vi "test13-Broadcast_Event.vi"(8 "error in (no error)":errorcluster, 11 "TestCase in":refnum<class "testcase-CSMGlobalLog.lvclass">) -> (0 "error out":errorcluster, 3 "TestCase out":refnum<class "testcase-CSMGlobalLog.lvclass">)   [LabVIEW 2017, in "testcase-CSMGlobalLog.lvclass"]
uses:
  testcase-CSMGlobalLog.lvclass
  testcase-CSMGlobalLog.lvclass/testcase-CSMGlobalLog.ctl
  src/user.lib/_NEVSTOP/Communicable State Machine(CSM)/_Support/Typedef/_CSM_GlobalLog_MSG.ctl
  src/user.lib/_NEVSTOP/Communicable State Machine(CSM)/_Support/Typedef/_CSM_Response Source Message.ctl
  src/user.lib/_NEVSTOP/Communicable State Machine(CSM)/_Support/Typedef/_CSM_GlobalLog_MSG_TYPE.ctl
  c0dc643a-0362-49fc-99f4-5251266ba5a0.vi
  src/user.lib/_NEVSTOP/Communicable State Machine(CSM)/_Support/GlobalEvent/GEvt-Generate with Rule Check.vi
  src/user.lib/_NEVSTOP/Communicable State Machine(CSM)/AdvanceAPI/CSM - Convert Error to Argument.vi
  src/user.lib/_NEVSTOP/Communicable State Machine(CSM)/AdvanceAPI/CSM - Make String Arguments Safe.vi
  src/user.lib/_NEVSTOP/Communicable State Machine(CSM)/AdvanceAPI/CSM - Keywords.vi
  src/user.lib/_NEVSTOP/Communicable State Machine(CSM)/_Support/GlobalEvent/Cache-GEvt Refs.vi
  src/user.lib/_NEVSTOP/Communicable State Machine(CSM)/_Support/GlobalEvent/LogFilter/LogFilter - Check.vi
  src/user.lib/_NEVSTOP/Communicable State Machine(CSM)/_Support/GlobalEvent/LogFilter/LogFilter.lvclass
  <vilib>/addons/_JKI Toolkits/VI Tester/TestCase.llb/TestCase.lvclass
  src/user.lib/_NEVSTOP/Communicable State Machine(CSM)/Communicable State Machine.lvlib
  CSM/CSM-Testcase.lvlib
  C:/Program Files (x86)/National Instruments/LabVIEW 2017/vi.lib/addons/_JKI Toolkits/VI Tester/TestCase.llb/TestCase.lvclass
panel:
  out "String cache each loop":string
  out "LoopCount":i32
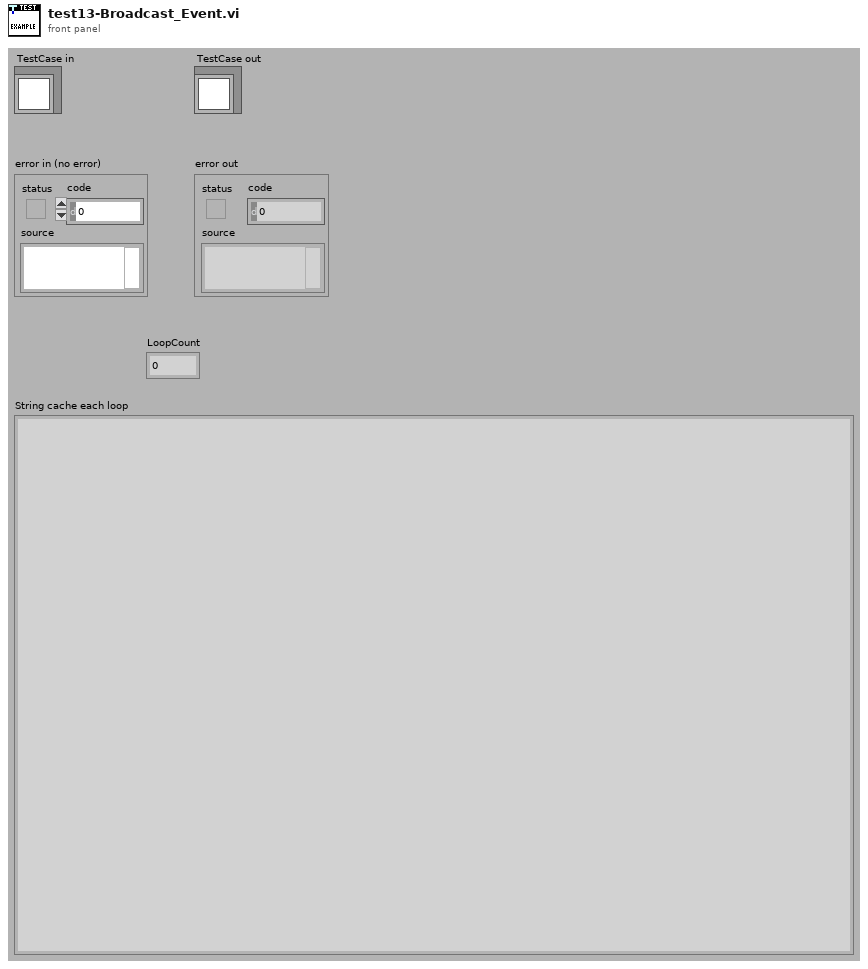
[diagram p1: front panel]
types:
  T1 = typedef "Communicable State Machine.lvlib/_CSM_GlobalLog_MSG.ctl" = cluster{"Name (\"\" to Use UUID)":string, "Current State":string, "Arguments":string, "Source Message":T2, "Source Module":string, "Complete(T)/Start(F)":bool, "LogType":T3, "Time Stamp":timestamp}
  T2 = typedef "Communicable State Machine.lvlib/_CSM_Response Source Message.ctl" = cluster{"‘State":string, "’Arguments":string, "’Error":errorcluster}
  T3 = typedef "Communicable State Machine.lvlib/_CSM_GlobalLog_MSG_TYPE.ctl" = enum16{"User Log", "State Change", "Status", "Interrupt", "Register", "Unregister", "Error Log", "Module Created", "Module Destroyed", "Async Message", "No-Rep Async Message", "Sync Message"}
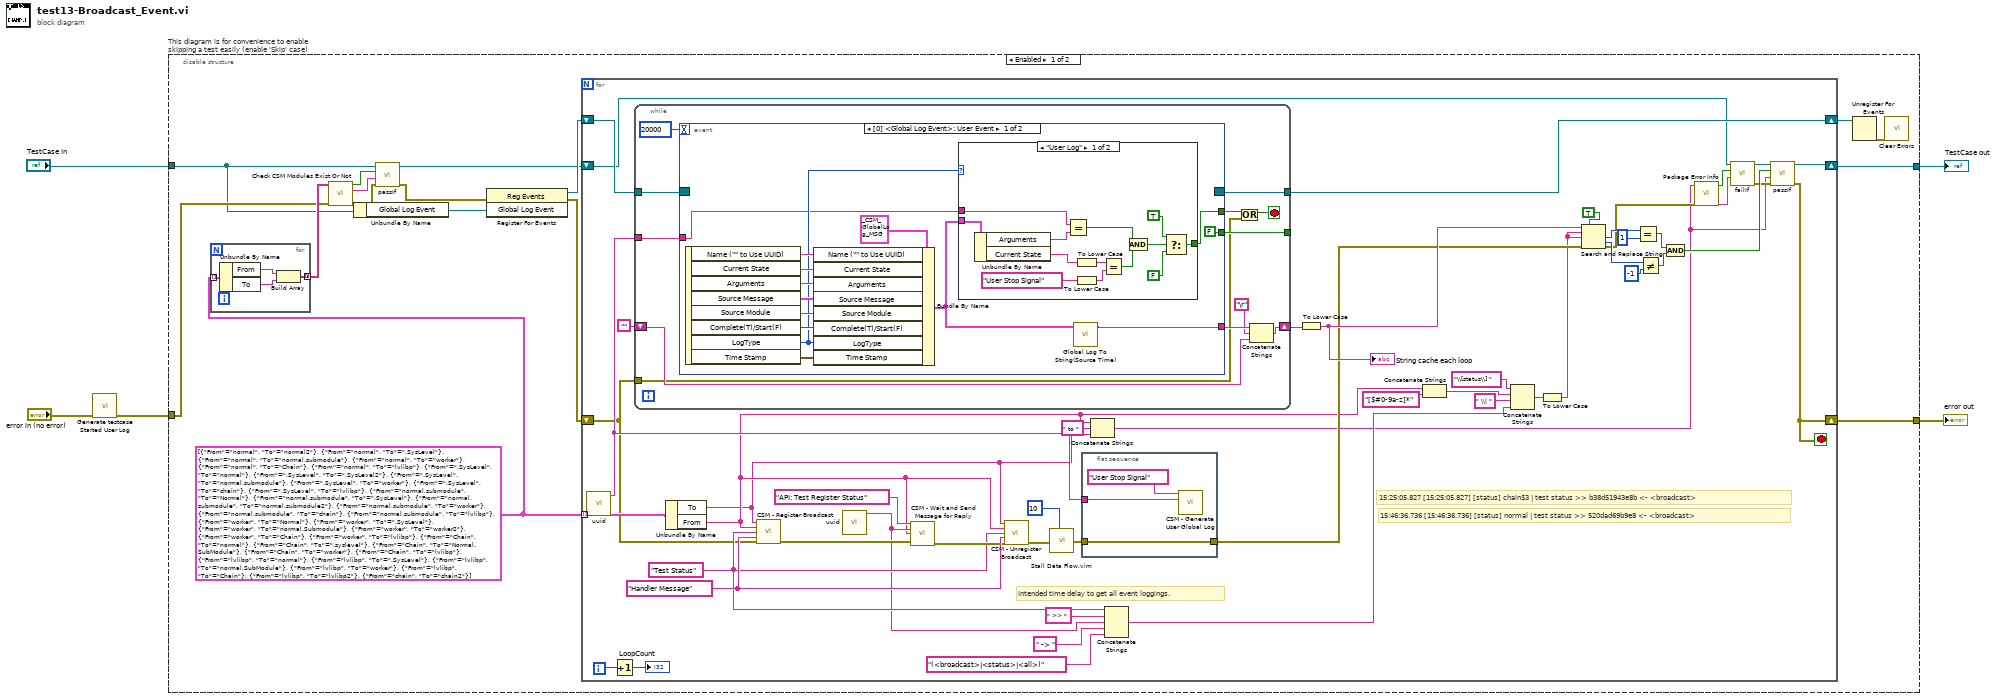
[diagram p0: block diagram]
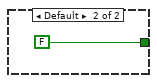
[diagram p2: hidden frame]
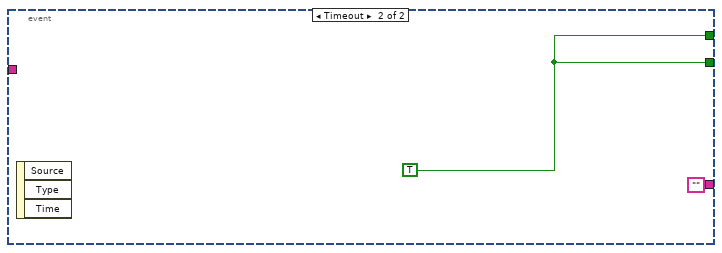
[diagram p3: hidden frame]
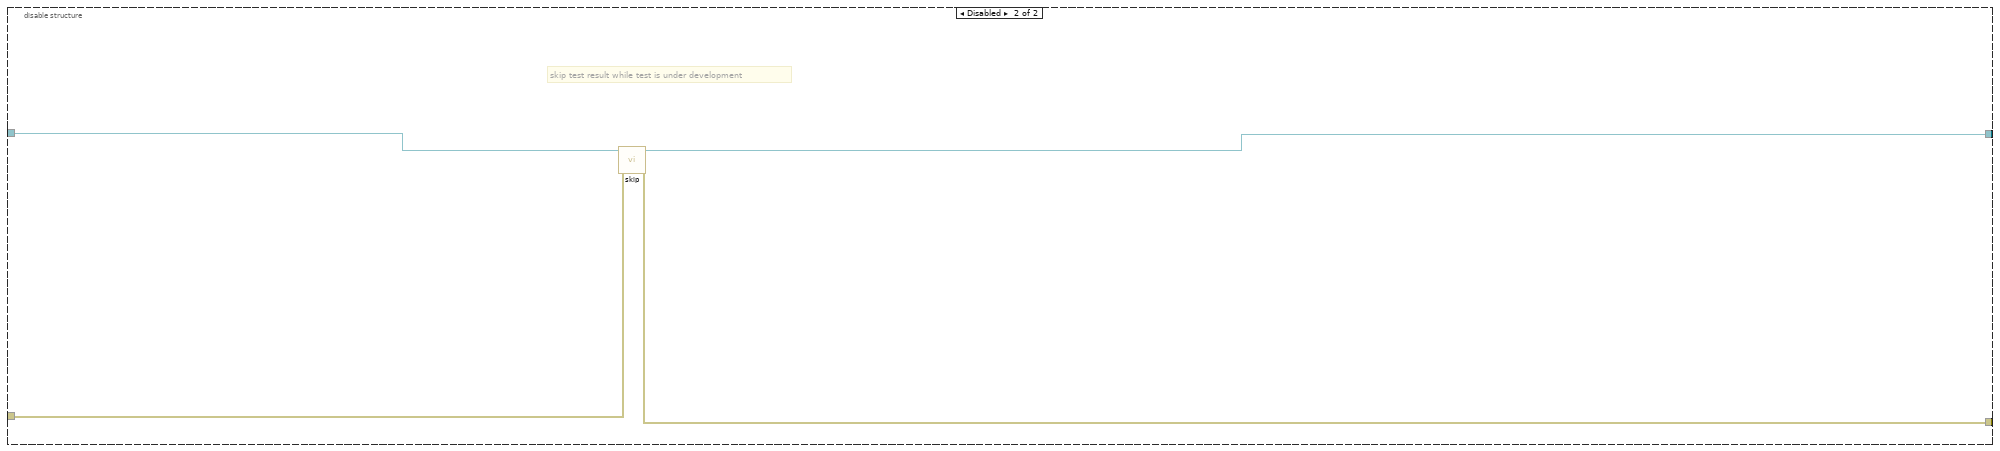
[diagram p4: hidden frame]
diagram:
  n1 = call "Generate testcase Started User Log.vi"("Error In"="error in (no error)") -> ("error out"=w1:errorcluster)  [unwired: 10 in]
  n2 = disable-structure "This diagram is for convenience to enable skipping a test easily (enable 'Skip' case)" shown="Enabled" {
    disable-tunnel: "TestCase in" -> [w7 w124]
    disable-tunnel: [w17 w122] -> w2
    disable-tunnel: [w16 w123] -> w4
    disable-tunnel: w1 -> [w10 w121]
    frame Enabled {
      w11 = cluster{"From":string, "To":string}[] [{"From"="normal", "To"="normal2"}, {"From"="normal", "To"=".SysLevel"}, {"From"="normal", "To"="normal.submodule"}, {"From"="normal", "To"="worker"}, {"From"="normal", "To"="Chain"}, {"From"="normal", "To"="lvlibp"}, {"From"=".SysLevel", "To"="normal"}, {"From"=".SysLevel", "To"=".SysLevel2"}, {"From"=".SysLevel", "To"="normal.submodule"}, {"From"=".SysLevel", "To"="worker"}, {"From"=".SysLevel", "To"="chain"}, {"From"=".SysLevel", "To"="lvlibp"}, {"From"="normal.submodule", "To"="Normal"}, {"From"="normal.submodule", "To"=".SysLevel"}, {"From"="normal.submodule", "To"="normal.submodule2"}, {"From"="normal.submodule", "To"="worker"}, {"From"="normal.submodule", "To"="chain"}, {"From"="normal.submodule", "To"="lvlibp"}, {"From"="worker", "To"="Normal"}, {"From"="worker", "To"=".SysLevel"}, {"From"="worker", "To"="normal.Submodule"}, {"From"="worker", "To"="worker2"}, {"From"="worker", "To"="Chain"}, {"From"="worker", "To"="lvlibp"}, {"From"="Chain", "To"="normal"}, {"From"="Chain", "To"=".syslevel"}, {"From"="Chain", "To"="Normal.SubModule"}, {"From"="Chain", "To"="worker"}, {"From"="Chain", "To"="lvlibp"}, {"From"="lvlibp", "To"="normal"}, {"From"="lvlibp", "To"=".SysLevel"}, {"From"="lvlibp", "To"="normal.SubModule"}, {"From"="lvlibp", "To"="worker"}, {"From"="lvlibp", "To"="Chain"}, {"From"="lvlibp", "To"="lvlibp2"}, {"From"="chain", "To"="chain2"}]
      n3 = for {
        tunnel: w11 -> [w25] mode=indexing
        tunnel: [w22] -> w14 mode=concatenating
        n4 = Unbundle By Name(w25) -> ("From"=w24:string, "To"=w23:string)
        n5 = Build Array(w24, w23) -> (w22:string[])
      }
      n6 = call "Check CSM Modules Exist Or Not.vi"("error in"=w10, "CSM names in"=w14) -> ("error out"=w12:errorcluster, "Debug string"=w13:string, "All Modules Exist?"=w15:bool)  [unwired: 7 in]
      n7 = Unbundle By Name(w7) -> ("Global Log Event"=w21:refnum<user-event>)
      n8 = call-dynamic "passIf.vi"("error in (no error)"=w12, "message (\"\")"=w13, "pass"=w15, "TestCase in"=w7) -> ("error out"=w8:errorcluster, "TestCase out"=w9:refnum<class "testcase-CSMGlobalLog.lvclass">)  [unwired: 6 in]
      n9 = register-events(error in=w8, w21) -> (reference out=w20:refnum<event-registration>, error out=w18:errorcluster)  [unwired: 1 in]
      n10 = for {
        shift-right: [w74] -> w19
        shift-left: w20 -> [w75]
        shift-right: [w71] -> w16
        shift-left: w18 -> [w36]
        tunnel: w11 -> [w50] mode=indexing
        shift-right: [w73] -> w17
        shift-left: w9 -> [w34]
        i -> [w60]
        stop <- w71 stop-if-true
        w55 = "Handler Message" ("API (If \"\", Same as Trigger)")
        w46 = "Test Status" ("Trigger")
        # "15:46:36.736 [15:46:36.736] [status] normal | test status >> 520dad69b9e8 <- <broadcast>"
        # "15:25:05.827 [15:25:05.827] [status] chain$3 | test status >> b38d51943e8b <- <broadcast>"
        # "Intended time delay to get all event loggings."
        n11 = call "uuid.vi"() -> ("UUID"=w61:string)  [unwired: 11 in]
        n12 = Increment(x=w60) -> (x+1=→"LoopCount":i32)
        n13 = while {
          tunnel: w75 -> [w90]
          tunnel: [w89] -> w74
          shift-right: [w82] -> w56
          shift-left: "" -> [w85]
          tunnel: w61 -> [w87]
          tunnel: [w86] -> _
          tunnel: w36 -> [w79]
          stop <- w81 stop-if-true
          n14 = event shown="[0] <Global Log Event>: User Event" {
            selector: w90 -> [_ _]
            dyn-events: [_ _] -> w89
            timeout: 20000 -> [_ _]
            tunnel: [w91 ""] -> w84
            tunnel: [w93 w120] -> w80
            tunnel: w87 -> [w94 _]
            tunnel: [FALSE ("Stop") w120] -> w86
            event User Event {
              n15 = event-data() -> ("Name (\"\" to Use UUID)"=w103:string, "Current State"=w102:string, "Arguments"=w101:string, "Source Message"=w100:T2, "Source Module"=w99:string, "Complete(T)/Start(F)"=w98:bool, "LogType"=w95:T3, "Time Stamp"=w97:timestamp)  [unwired: 1 in]
              n16 = Bundle By Name(cluster=T1 {"Name (\"\" to Use UUID)"="", "Current State"="", "Arguments"="", "Source Message"={"‘State"="", "’Arguments"="", "’Error"={"status"=FALSE, "code"=0, "source"=""}}, "Source Module"="", "Complete(T)/Start(F)"=FALSE, "LogType"=enum."State Change", "Time Stamp"=timestamp(0 s since 1904-01-01)} ("Cross CSM Data"), "Name (\"\" to Use UUID)"=w103, "Current State"=w102, "Arguments"=w101, "Source Message"=w100, "Source Module"=w99, "Complete(T)/Start(F)"=w98, "LogType"=w95, "Time Stamp"=w97) -> (w92:T1)
              n17 = case shown="\"User Log\"" w95 {
                tunnel: w92 -> [w117 _]
                tunnel: w94 -> [w116 _]
                tunnel: [w105 FALSE] -> w93
                frame "User Log" {
                  n18 = Unbundle By Name(w117) -> ("Arguments"=w115:string, "Current State"=w114:string)
                  n19 = Equal?(x=w116, y=w115) -> (x = y?=w109:bool)
                  n20 = To Lower Case(string=w114) -> (all lower case string=w113:string)
                  n21 = To Lower Case(string="User Stop Signal" ("Log")) -> (all lower case string=w111:string)
                  n22 = Equal?(x=w113, y=w111) -> (x = y?=w110:bool)
                  n23 = And(x=w109, y=w110) -> (x .and. y?=w108:bool)
                  n24 = Select(t=TRUE, s=w108, f=FALSE) -> (s? t:f=w105:bool)
                }
                frame Default {
                }
              }
              n25 = call "Global Log To String(Source Time).vi"("Log"=w92) -> ("Log String"=w91:string)  [unwired: 9 in]
            }
            event Timeout {
              w120 = TRUE ("Stop")
              n26 = event-data() -> ()  [unwired: 1 in, 3 out]
            }
          }
          n27 = Or(x=w80, y=w79) -> (x .or. y?=w81:bool)
          n28 = Concatenate Strings(w84, "\r", w85) -> (w82:string)
        }
        n29 = Unbundle By Name(w50) -> ("To"=w29:string, "From"=w30:string)
        n30 = call "CSM - Register Broadcast.vi"("CSM Name(Empty for Broadcast Event)"=w29, "Source CSM Name (* as Default)"=w30, "Trigger"=w46, "API (If \"\", Same as Trigger)"=w55, "Error In"=w36) -> ("error out"=w52:errorcluster)  [unwired: 9 in, 1 out]
        n31 = call "uuid.vi"() -> ("UUID"=w45:string)  [unwired: 11 in]
        n32 = call "CSM - Wait and Send Message for Reply.vi"("State"="API: Test Register Status", "Arguments (\"\")"=w45, "Target Module"=w30, "Error In (No Error)"=w52) -> ("error out"=w53:errorcluster)  [unwired: 8 in, 3 out]
        n33 = call "CSM - Unregister Broadcast.vi"("CSM Name(Empty for Broadcast Event)"=w29, "Source CSM Name (* as Default)"=w30, "Trigger"=w46, "API (\"*\" as Default)"=w55, "Error In"=w53) -> ("error out"=w51:errorcluster)  [unwired: 9 in, 1 out]
        n34 = call "Stall Data Flow.vim"("value in"=w51, "milliseconds to wait"=u32 10) -> ("value out"=w62:errorcluster)  [unwired: 1 out]
        n35 = flat-sequence {
          tunnel: w61 -> [w77]
          tunnel: w62 -> [w76]
          tunnel: [w76] -> w57
          frame #0 {
            n36 = call "CSM - Generate User Global Log.vi"("Arguments"=w77, "Log"="User Stop Signal") -> ()  [unwired: 9 in, 1 out]
          }
        }
        n37 = Concatenate Strings(w30, " to " ("string"), w29) -> (w26:string)
        n38 = Concatenate Strings(w46, " >> " ("string"), w45, " -> " ("string"), "(<broadcast>|<status>|<all>)" ("search string")) -> (w38:string)
        n39 = To Lower Case(string=w56) -> (all lower case string=w58:string)
        "String cache each loop" <- w58
        n40 = Concatenate Strings(w30, "[$#0-9a-z]*" ("string")) -> (w39:string)
        n41 = Concatenate Strings("\\[status\\] " ("regular expression"), w39, " \\| " ("string"), w38) -> (w42:string)
        n42 = To Lower Case(string=w42) -> (all lower case string=w37:string)
        n43 = Search and Replace String(replace all?=TRUE ("replace all? (F)"), input string=w58, search string=w37, replace string=w37, error in=w57) -> (number of replacements=w67:i32, offset past replacement=w68:i32, error out=w31:errorcluster)  [unwired: 3 in, 1 out]
        n44 = Equal?(x=w67, y=1) -> (x = y?=w69:bool)
        n45 = Not Equal?(x=w68, y=-1) -> (x != y?=w70:bool)
        n46 = And(x=w69, y=w70) -> (x .and. y?=w44:bool)
        n47 = call "Package Error Info.vi"("error in"=w31, "String in"=w26) -> ("packed error info out"=w32:string, "error status"=w35:bool)  [unwired: 8 in]
        n48 = call-dynamic "failIf.vi"("message (\"\")"=w32, "fail"=w35, "TestCase in"=w34) -> ("error out"=w27:errorcluster, "TestCase out"=w33:refnum<class "testcase-CSMGlobalLog.lvclass">)  [unwired: 7 in]
        n49 = call-dynamic "passIf.vi"("error in (no error)"=w27, "message (\"\")"=w26, "pass"=w44, "TestCase in"=w33) -> ("error out"=w71:errorcluster, "TestCase out"=w73:refnum<class "testcase-CSMGlobalLog.lvclass">)  [unwired: 6 in]
      }
      n50 = Unregister For Events(event registration refnum=w19) -> (error out=w6:errorcluster)  [unwired: 1 in]
      n51 = call <vilib>:"Clear Errors.vi"("error in (no error)"=w6) -> ()  [unwired: 5 in, 2 out]
    }
    frame Disabled {
      # "skip test result while test is under development"
      n52 = call <vilib>:"skip.vi"("error in (no error)"=w121, "TestCase in"=w124) -> ("error out"=w123:errorcluster, "TestCase out"=w122:refnum<class "testcase-CSMGlobalLog.lvclass">)  [unwired: 8 in]
    }
  }
  "error out" <- w4
  "TestCase out" <- w2
